vi "Compass on new GIC parallel 2.vi"(11 "GIC Input 2":T1={"     Use ?\nOff       On"=[FALSE, TRUE, FALSE, TRUE], "Mode:"=FALSE, "Extra Port"="", "Hokuyo Port"="COM7", "Tx Prop  Port"="COM6", "Compass Port"="", "GPS Port"="", "Num of WPs"=0, "WP Lats and Longs"={"WP Lats"=[], "WP Longs"=[]}, "Obst Lats and Longs"={"Obst Lats"=[], "Obst Longs"=[]}, "Parameters"=[], "GPS Data"=[], "Compass"=0.0, "LMS Vector"=[], "Vision Vector"=[], "Direction Cmd"=0.0, "Speed Cmd"=0.0, "WP Vector"=[], "WP Number"=0, "Extra"=0, "SW Map"=[], "Path Cluster"={"Path x node"=[], "Path y node"=[]}, "Sim Course"=[]} {"Obst Lats and Longs"."Obst Longs" format="%#_8g"; "Obst Lats and Longs"."Obst Lats" format="%#_8g"}) -> (3 "GIC Output 2":T1={"     Use ?\nOff       On"=[FALSE, TRUE, FALSE, TRUE], "Mode:"=FALSE, "Extra Port"="", "Hokuyo Port"="COM7", "Tx Prop  Port"="COM6", "Compass Port"="", "GPS Port"="", "Num of WPs"=0, "WP Lats and Longs"={"WP Lats"=[], "WP Longs"=[]}, "Obst Lats and Longs"={"Obst Lats"=[], "Obst Longs"=[]}, "Parameters"=[], "GPS Data"=[], "Compass"=0.0, "LMS Vector"=[], "Vision Vector"=[], "Direction Cmd"=0.0, "Speed Cmd"=0.0, "WP Vector"=[], "WP Number"=0, "Extra"=0, "SW Map"=[], "Path Cluster"={"Path x node"=[], "Path y node"=[]}, "Sim Course"=[]} {"Obst Lats and Longs"."Obst Longs" format="%#_8g"; "Obst Lats and Longs"."Obst Lats" format="%#_8g"})   [LabVIEW 2014]
uses:
  Global_vars.vi
panel:
  out "compass out":dbl
  # "Compass on new GIC parallel 2"
  # "Compass on New GIC A"
  # "Input:"
  # "Output:"
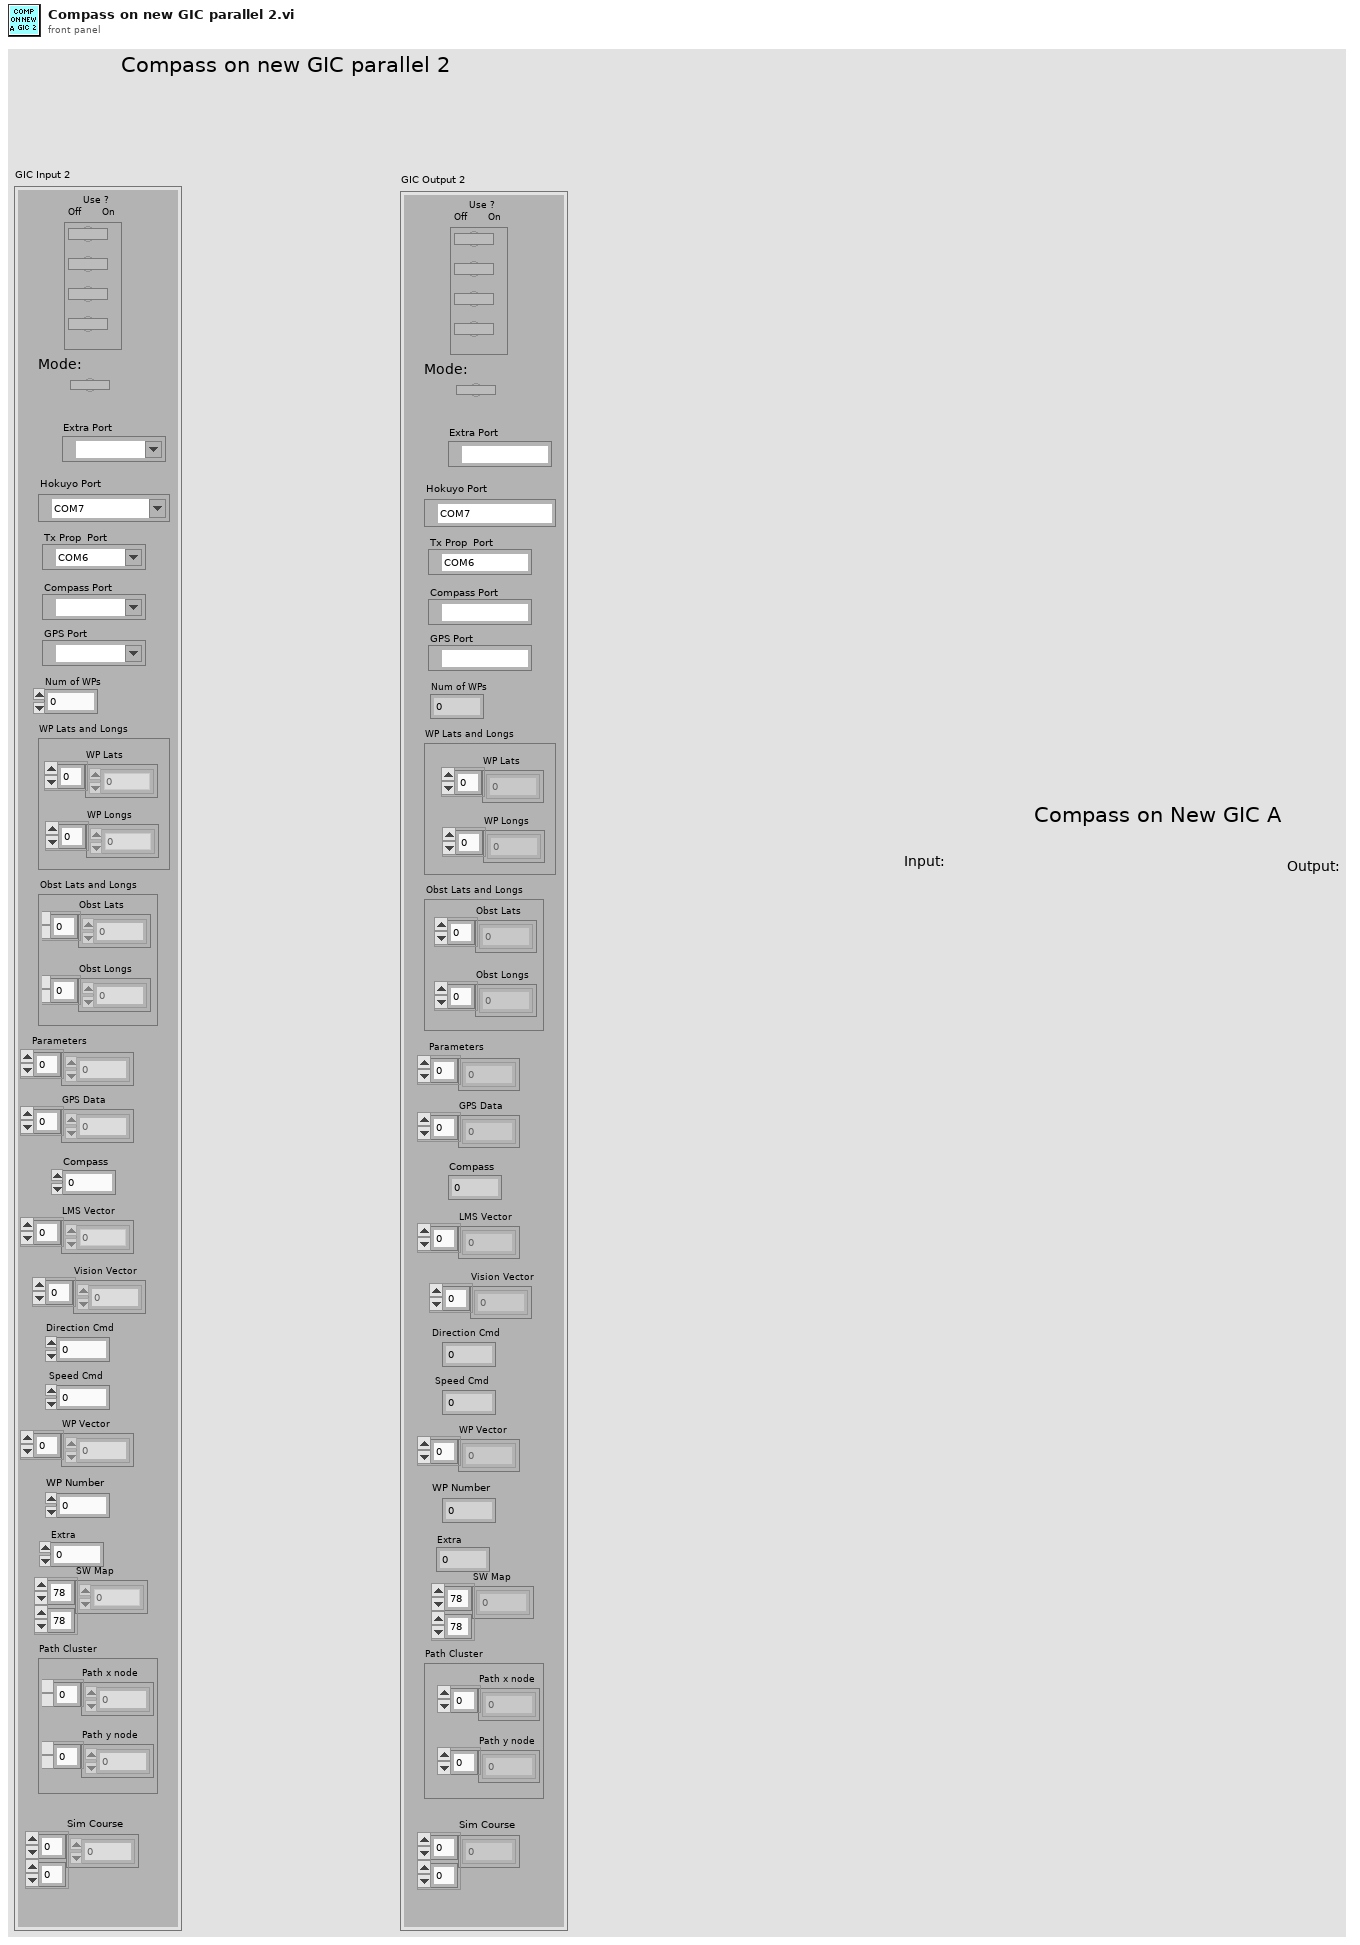
[diagram p1: front panel]
types:
  T1 = cluster{"     Use ?\nOff       On":bool[], "Mode:":bool, "Extra Port":refnum<visa-resource-name>, "Hokuyo Port":refnum<visa-resource-name>, "Tx Prop  Port":refnum<visa-resource-name>, "Compass Port":refnum<visa-resource-name>, "GPS Port":refnum<visa-resource-name>, "Num of WPs":i16, "WP Lats and Longs":cluster{"WP Lats":dbl[], "WP Longs":dbl[]}, "Obst Lats and Longs":cluster{"Obst Lats":dbl[], "Obst Longs":dbl[]}, "Parameters":dbl[], "GPS Data":dbl[], "Compass":dbl, "LMS Vector":dbl[], "Vision Vector":dbl[], "Direction Cmd":dbl, "Speed Cmd":dbl, "WP Vector":dbl[], "WP Number":i32, "Extra":i16, "SW Map":i32[][], "Path Cluster":cluster{"Path x node":dbl[], "Path y node":dbl[]}, "Sim Course":i8[][]}
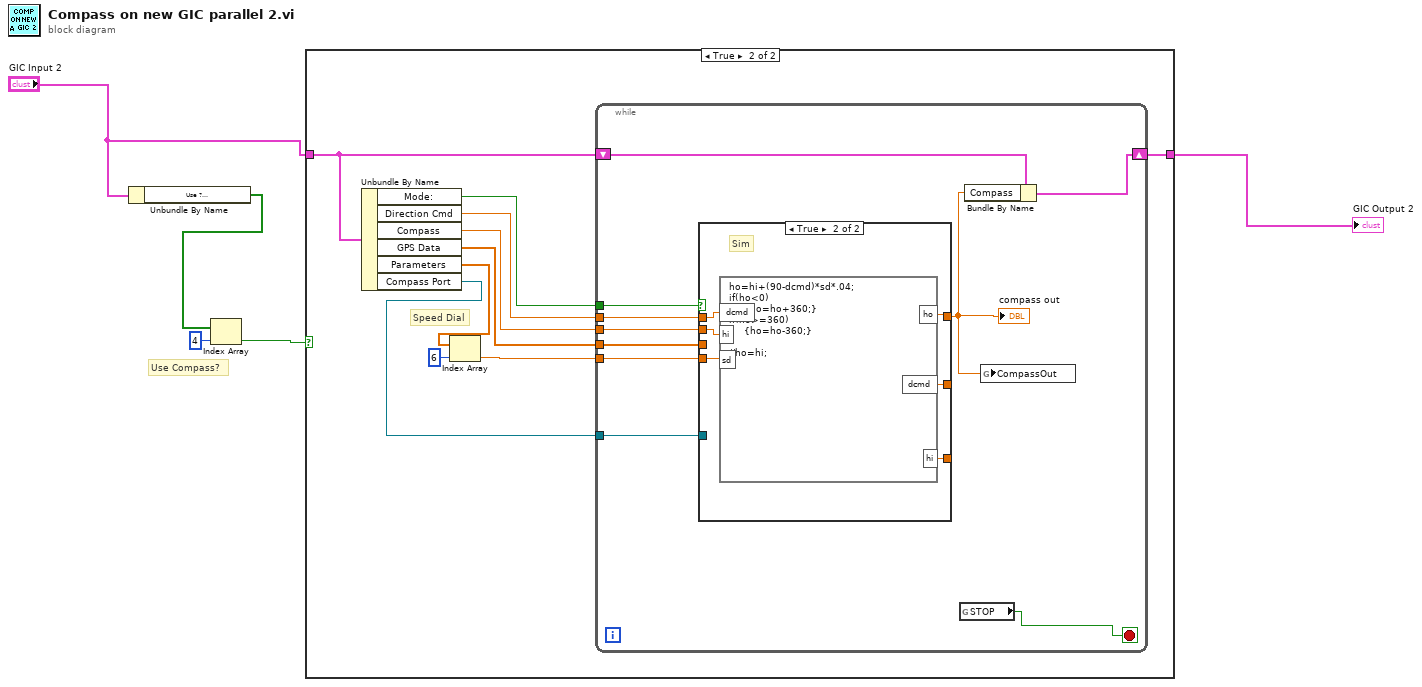
[diagram p0: block diagram]
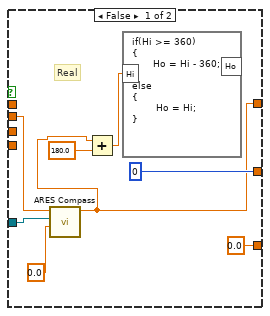
[diagram p3: hidden frame]
diagram:
  # "Use Compass?"
  n1 = Unbundle By Name("GIC Input 2") -> ("Use ?\nOff       On"=w5:bool[])
  n2 = Index Array(array=w5, index=4) -> (element=w3:bool)
  n3 = case shown="True" w3 {
    tunnel: "GIC Input 2" -> [w6 w7]
    tunnel: [w6 w8] -> w1
    frame False {
    }
    frame True {
      # "Speed Dial"
      n4 = Unbundle By Name(w7) -> ("Mode:"=w15:bool, "Direction Cmd"=w11:dbl, "Compass"=w10:dbl, "GPS Data"=w16:dbl[], "Parameters"=w14:dbl[], "Compass Port"=w9:refnum<visa-resource-name>)
      n5 = Index Array(array=w14, index=6) -> (element=w12:dbl)
      n6 = while {
        tunnel: w16 -> [w26]
        tunnel: w15 -> [w25]
        tunnel: w12 -> [w24]
        tunnel: w11 -> [w23]
        tunnel: w10 -> [w22]
        tunnel: w9 -> [w21]
        shift-right: [w17] -> w8
        shift-left: w7 -> [w18]
        stop <- w19 stop-if-true
        n7 = case shown="True" w25 {
          tunnel: w23 -> [_ w39]
          tunnel: w22 -> [w32 w38]
          tunnel: [w27 w40] -> w20
          tunnel: w26 -> [_ _]
          tunnel: w24 -> [_ w37]
          tunnel: [0 w36] -> _
          tunnel: [0.0 ("hi") w35] -> _
          tunnel: w21 -> [w31 _]
          frame False {
            # "Real"
            n8 = call "ARES Compass.vi"("Input time of last compass read"=0.0, "Compass Com Port"=w31, "Compass In"=w32) -> ("Compass Out"=w27:dbl)  [unwired: 6 in, 1 out]
            n9 = Add(x=w27, y=180.0) -> (x+y=w28:dbl)
            n10 = formula code="if(Hi >= 360)\n{\n       Ho = Hi - 360;\n}\nelse\n{\n        Ho = Hi;\n}"("Hi"=w28) -> ()  [unwired: 1 out]
          }
          frame True {
            # "Sim"
            n11 = formula code="ho=hi+(90-dcmd)*sd*.04;\nif(ho<0)\n     {ho=ho+360;}\nif(ho>=360)\n     {ho=ho-360;}\n\n//ho=hi;"("dcmd"=w39, "hi"=w38, "sd"=w37) -> ("ho"=w40:dbl, "dcmd"=w36:dbl, "hi"=w35:dbl)
          }
        }
        "compass out" <- w20
        n12 = global read "Global_vars.vi" "STOP"() -> (w19:bool)
        n13 = Bundle By Name(cluster=w18, "Compass"=w20) -> (w17:T1)
        n14 = global write "Global_vars.vi" "CompassOut"(w20) -> ()
      }
    }
  }
  "GIC Output 2" <- w1
